vi "DD Enabler.vi"() -> ()   [LabVIEW 2011]
uses:
  <vilib>/Utility/traverseref.llb/TRef TravTarget.ctl
  <vilib>/Utility/traverseref.llb/VI Scripting - Traverse.lvlib
panel:
  in  "Active Frame":i16
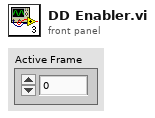
[diagram p1: front panel]
types:
  T1 = typedef "TRef TravTarget.ctl" = enum16{"FP", "BD", "Other"}
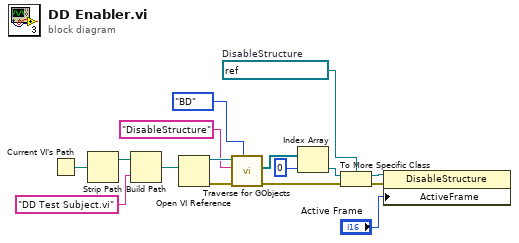
[diagram p0: block diagram]
diagram:
  w10 = refnum<vi> refnum  # DisableStructure
  n1 = Current VI's Path() -> (path=w4:path)
  n2 = Strip Path(path=w4) -> (stripped path=w3:path)  [unwired: 1 out]
  n3 = Build Path(base path=w3, name or relative path="DD Test Subject.vi") -> (appended path=w1:path)
  n4 = Open VI Reference(vi path=w1) -> (vi reference=w16:refnum<vi>, error out=w6:errorcluster)  [unwired: 5 in]
  n5 = call <vilib>:"Traverse for GObjects.vi"("Traverse Target"=TRef_TravTarget."BD", "error in (no error)"=w6, "Class Name"="DisableStructure", "VI Refnum"=w16) -> ("error out"=w7:errorcluster, "References"=w13:refnum<vi>[])  [unwired: 4 in, 2 out]
  n6 = Index Array(array=w13, index=0) -> (element=w11:refnum<vi>)
  n7 = To More Specific Class(target class=w10, reference=w11, error in=w7) -> (specific class reference=w9:refnum<vi>, error out=w8:errorcluster)
  n8 = property class="DisableStructure"(reference=w9, error in=w8, "ActiveFrame"="Active Frame") -> ()  [unwired: 2 out]
